vi "Read GaugeController Obj.vi"(8 "error in (no error)":errorcluster, 11 "GaugeController Configuration in":refnum<class "GaugeController Configuration.lvclass">) -> (0 "error out":errorcluster, 2 "GaugeController.lvclass":refnum<class "GaugeController.lvclass">, 3 "GaugeController Configuration out":refnum<class "GaugeController Configuration.lvclass">)   [LabVIEW 2016, in "Hardware.lvlib" / "GaugeController.lvlib" / "GaugeController Configuration.lvclass"]
uses:
  <userlib>/Common Components/Hardware/GaugeController/GaugeController Config/GaugeController Configuration.lvclass
  <userlib>/Common Components/Hardware/GaugeController/GaugeController/GaugeController.lvclass
  <userlib>/Common Components/Hardware/GaugeController/GaugeController Config/GaugeController Configuration.lvclass/GaugeController Configuration.ctl
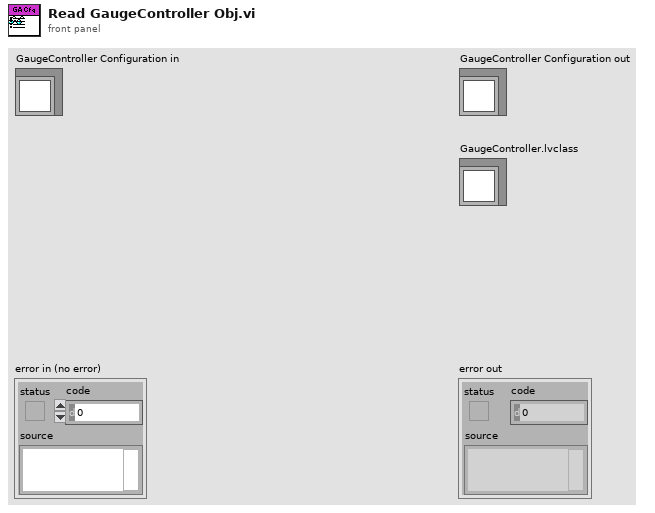
[diagram p1: front panel]
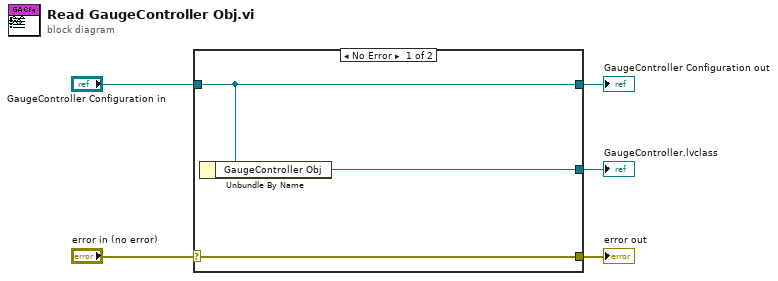
[diagram p0: block diagram]
diagram:
  n1 = case shown="No Error" "error in (no error)" {
    selector: "error in (no error)" -> [w8 w9]
    tunnel: [w8 w9] -> w4
    tunnel: [w7 w10] -> w2
    tunnel: "GaugeController Configuration in" -> [w7 w10]
    tunnel: [w6 _] -> w1
    frame No Error {
      n2 = Unbundle By Name(w7) -> ("GaugeController Obj"=w6:refnum<class "GaugeController.lvclass">)
    }
    frame Error {
    }
  }
  "error out" <- w4
  "GaugeController Configuration out" <- w2
  "GaugeController.lvclass" <- w1
